vi "read and write file.vi"(6 "data to write":string[][](array[string])=[["admin", "password"], ["oprator", "text"], ["oprator1", "text1"], ["oprator2", "text2"], ["oprator3", "text3"]], 10 "Path":path=path "E:/labview code/project user login/test1.txt", 11 "Enum":enum16{"write", "read"}(ring)) -> (3 "output data":string[][](array[string]))   [LabVIEW 2015]
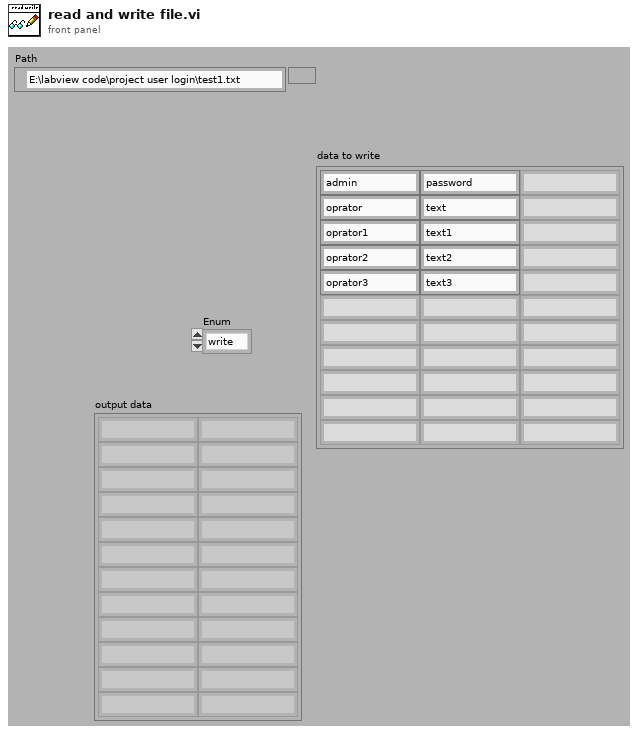
[diagram p1: front panel]
types:
  T1 = enum16{"open", "replace", "create", "open or create", "replace or create", "replace or create with confirmation"}
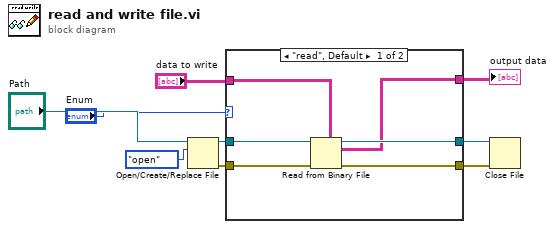
[diagram p0: block diagram]
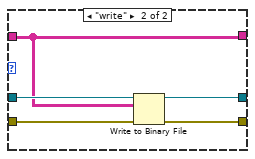
[diagram p2: hidden frame]
diagram:
  n1 = Open/Create/Replace File(file path (use dialog)="Path", operation (0:open)=T1."open") -> (refnum out=w7:refnum<file>, error out=w4:errorcluster)  [unwired: 4 in, 1 out]
  n2 = case shown="\"read\", Default" "Enum" {
    tunnel: w7 -> [w15 w20]
    tunnel: [w14 w19] -> w6
    tunnel: "data to write" -> [w13 w18]
    tunnel: [w12 w18] -> w2
    tunnel: w4 -> [w11 w17]
    tunnel: [w10 w16] -> w3
    frame "read", Default {
      n3 = Read from Binary File(5:w13, 8:w11, 11:w15) -> (0:w10:errorcluster, 2:w12:string[][], 3:w14:refnum<file>)  [unwired: 3 in, 1 out]
    }
    frame "write" {
      n4 = Write to Binary File(file (use dialog)=w20, data=w18, error in=w17) -> (refnum out=w19:refnum<file>, error out=w16:errorcluster)  [unwired: 3 in, 1 out]
    }
  }
  "output data" <- w2
  n5 = Close File(refnum=w6, error in=w3) -> ()  [unwired: 2 out]
